vi "Hatch4barCollisionAvoidance.vi"(10 "Current4barSetpoint":dbl, 11 "Hatch Setpoint":dbl) -> (3 "Modified 4bar setpoint":dbl)   [LabVIEW 2018]
uses:
  Infrastructure/Constants.vi
  Robot Global Data.vi
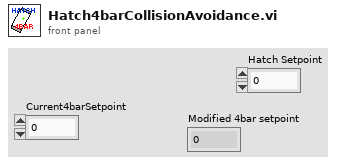
[diagram p1: front panel]
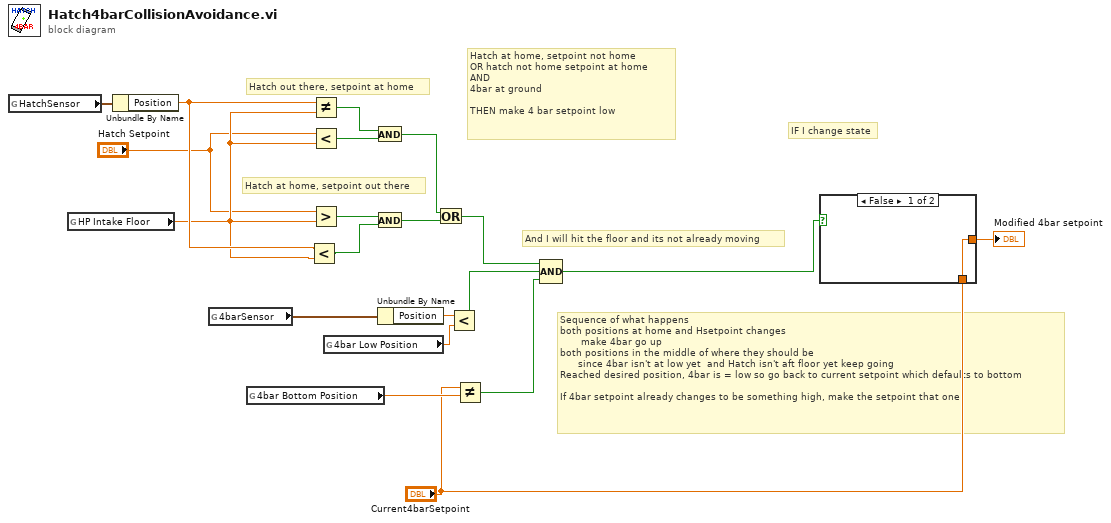
[diagram p0: block diagram]
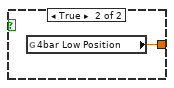
[diagram p2: hidden frame]
diagram:
  # "And I will hit the floor and its not already moving"
  # "IF I change state"
  # "Hatch out there, setpoint at home"
  # "Hatch at home, setpoint out there"
  # "Sequence of what happens\nboth positions at home and Hsetpoint changes\n       make 4bar go up\nboth positions in the middle of where they should be\n      since 4bar isn't at low yet  and Hatch isn't aft floor yet keep going\nReached desired position, 4bar is = low so go back to current setpoint which defaults to bottom\n\nIf 4bar setpoint already changes to be something high, make the setpoint that one"
  # "Hatch at home, setpoint not home\nOR hatch not home setpoint at home \nAND\n4bar at ground\n\nTHEN make 4 bar setpoint low"
  n1 = global read "Robot Global Data.vi" "HatchSensor"() -> (w17:cluster{"Position":dbl, "Velocity":dbl})
  n2 = global read "Constants.vi" "HP Intake Floor"() -> (w8:dbl)
  n3 = Unbundle By Name(w17) -> ("Position"=w10:dbl)
  n4 = global read "Robot Global Data.vi" "4barSensor"() -> (w14:cluster{"Position":dbl, "Velocity":dbl})
  n5 = global read "Constants.vi" "4bar Bottom Position"() -> (w4:dbl)
  n6 = Less?(x=w10, y=w8) -> (x < y?=w11:bool)
  n7 = Not Equal?(x=w10, y=w8) -> (x != y?=w16:bool)
  n8 = Less?(x="Hatch Setpoint", y=w8) -> (x < y?=w9:bool)
  n9 = Greater?(x="Hatch Setpoint", y=w8) -> (0:w19:bool)
  n10 = global read "Constants.vi" "4bar Low Position"() -> (w20:dbl)
  n11 = And(x=w16, y=w9) -> (x .and. y?=w15:bool)
  n12 = And(x=w19, y=w11) -> (x .and. y?=w18:bool)
  n13 = Unbundle By Name(w14) -> ("Position"=w13:dbl)
  n14 = Or(x=w15, y=w18) -> (x .or. y?=w6:bool)
  n15 = Less?(x=w13, y=w20) -> (x < y?=w5:bool)
  n16 = Not Equal?(x="Current4barSetpoint", y=w4) -> (x != y?=w3:bool)
  n17 = Compound Arithmetic op=AND(w6, w5, w3) -> (w2:bool)
  n18 = case shown="False" w2 {
    tunnel: [w21 w22] -> w12
    tunnel: "Current4barSetpoint" -> [w21 _]
    frame False {
    }
    frame True {
      n19 = global read "Constants.vi" "4bar Low Position"() -> (w22:dbl)
    }
  }
  "Modified 4bar setpoint" <- w12
